vi "deinitialize.vi"(0 "HGF_SVMonitor":refnum<class "HGF_SVMonitor.lvclass">, 5 "error in (no error)":errorcluster) -> (19 "error out":errorcluster)   [LabVIEW 2012, in "HGF_SV.lvlib" / "HGF_SVMonitor.lvclass"]
doc: "This is a dynamic dispatch VI. It can be overwritten by childclasses to release allocated recources."
uses:
  HGF_SVMonitor.lvclass
  HGF_Monitor/HGF_Monitor.lvclass
  HGF_SVMonitor.lvclass/HGF_SVMonitor.ctl
  HGF_BaseClasses/HGF_NetworkVisitor/HGF_NetworkVisitor.lvclass
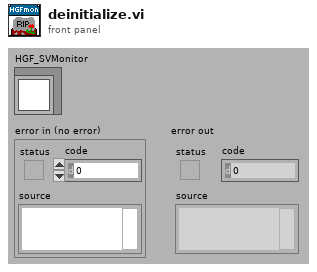
[diagram p1: front panel]
types:
  T1 = cluster{"registered Visitors":cluster{"HGF_NetworkVisitor":refnum<class "HGF_NetworkVisitor.lvclass">, "HGF_TriggeredEvent":refnum<class "HGF_TriggeredEvent.lvclass">}[], "last known data":variant, "Time Stamp":timestamp, "shared variable refnum in":refnum<k21>}[]
  T2 = cluster{"HGF_NetworkVisitor":refnum<class "HGF_NetworkVisitor.lvclass">, "HGF_TriggeredEvent":refnum<class "HGF_TriggeredEvent.lvclass">}[]
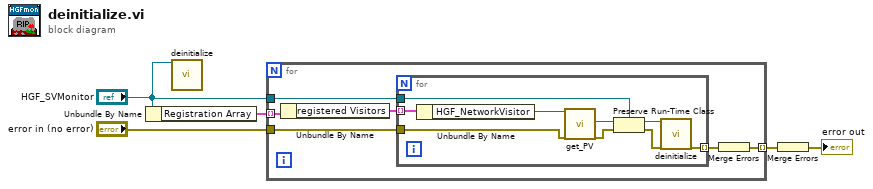
[diagram p0: block diagram]
diagram:
  n1 = Unbundle By Name("HGF_SVMonitor") -> ("Registration Array"=w5:T1)
  n2 = call-parent "deinitialize.vi"("HGF_Factory"="HGF_SVMonitor") -> ()  [unwired: 1 in, 18 out]
  n3 = for {
    tunnel: w5 -> [w11] mode=indexing
    tunnel: "error in (no error)" -> [w9]
    tunnel: [w7] -> w4 mode=indexing
    tunnel: "HGF_SVMonitor" -> [w6]
    n4 = Unbundle By Name(w11) -> ("registered Visitors"=w10:T2)
    n5 = for {
      tunnel: w10 -> [w20] mode=indexing
      tunnel: w9 -> [w14]
      tunnel: [w17] -> w8 mode=indexing
      tunnel: w6 -> [w15]
      n6 = Unbundle By Name(w20) -> ("HGF_NetworkVisitor"=w19:refnum<class "HGF_NetworkVisitor.lvclass">)
      n7 = call "get_PV.vi"("HGF_NetworkData"=w19, "error in (no error)"=w14) -> ("HGV_PVBase"=w18:refnum<class "HGF_PVBase.lvclass">, "error out"=w13:errorcluster)  [unwired: 16 out]
      n8 = Preserve Run-Time Class(object in=w18, error in=w13, 2:w15) -> (object out=w16:refnum<class "HGF_SVMonitor.lvclass">, error out=w12:errorcluster)
      n9 = call-parent "deinitialize.vi"("HGF_Factory"=w16, "error in (no error)"=w12) -> ("error out"=w17:errorcluster)  [unwired: 17 out]
    }
    n10 = Merge Errors(w8) -> (w7:errorcluster)
  }
  n11 = Merge Errors(w4) -> (→"error out":errorcluster)
